vi "http_request.vi"(8 "error in (no error)":errorcluster, 11 "url":string) -> (0 "error out":errorcluster)   [LabVIEW 2019]
uses:
  <vilib>/httpClient/LabVIEWHTTPClient.lvlib
panel:
  out "body":string
  out "headers":string
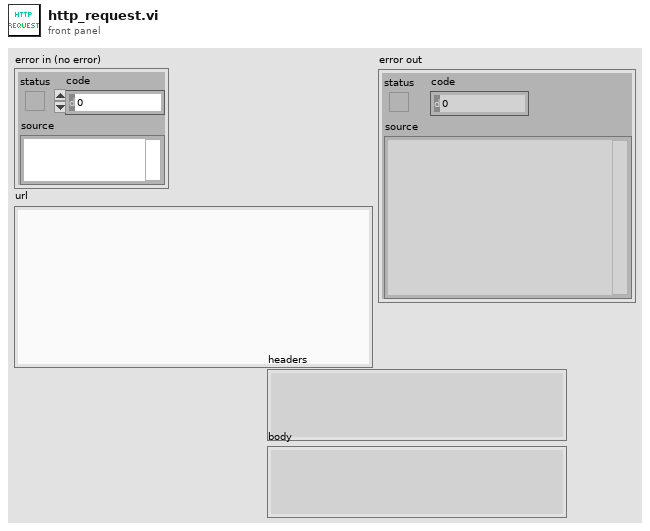
[diagram p1: front panel]
types:
  T1 = typedef "LabVIEWHTTPClient.lvlib/ClientHandle.ctl" = refnum<k1>
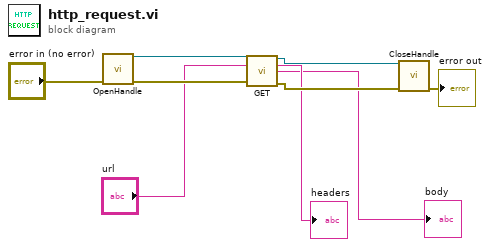
[diagram p0: block diagram]
diagram:
  n1 = call <vilib>:"OpenHandle.vi"("error in (no error)"="error in (no error)") -> ("client handle out"=w5:T1, "error out"=w7:errorcluster)  [unwired: 13 in]
  n2 = call <vilib>:"GET.vi"("client handle"=w5, "url"="url", "error in (no error)"=w7) -> ("client handle out"=w4:T1, "headers"=→"headers":string, "body"=→"body":string, "error out"=w6:errorcluster)  [unwired: 9 in]
  n3 = call <vilib>:"CloseHandle.vi"("client handle"=w4, "error in (no error)"=w6) -> ("error out"=→"error out":errorcluster)  [unwired: 13 in]
